vi "score target tracking.vi"() -> (0 "Boolean":bool)   [LabVIEW 2018]
uses:
  <vilib>/Rock Robotics/Network Tables/NT Write Number.vi
  <vilib>/Rock Robotics/Network Tables/NT Read Boolean.vi
  Robot Global Data.vi
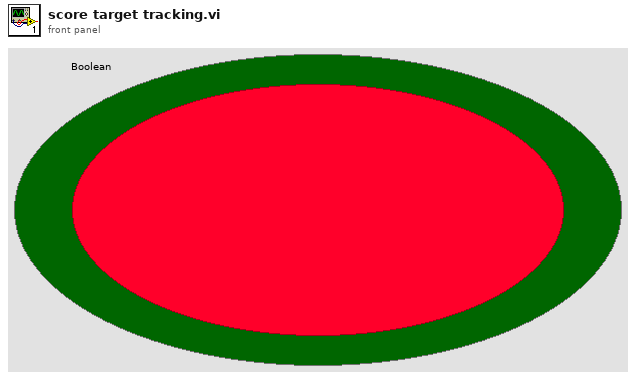
[diagram p1: front panel]
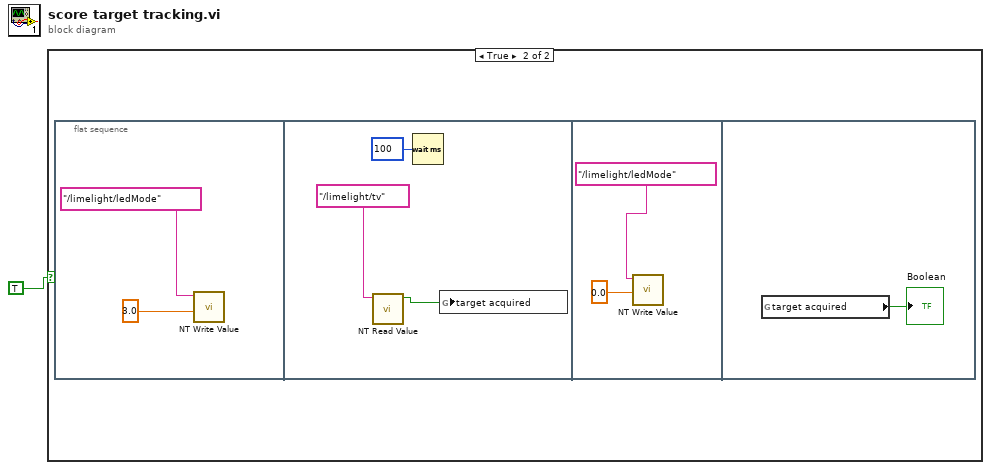
[diagram p0: block diagram]
diagram:
  n1 = case shown="True" TRUE {
    frame False {
    }
    frame True {
      n2 = flat-sequence {
        frame #0 {
          n3 = call-poly <vilib>:"NT Write Value.vi"("Numeric"=3.0, "Name"="/limelight/ledMode") -> ()  [unwired: 9 in, 1 out]
        }
        frame #1 {
          n4 = call-poly <vilib>:"NT Read Value.vi"("Name"="/limelight/tv") -> ("Boolean"=w5:bool)  [unwired: 9 in, 1 out]
          n5 = Wait (ms)(milliseconds to wait=u32 100) -> ()  [unwired: 1 out]
          n6 = global write "Robot Global Data.vi" "target acquired"(w5) -> ()
        }
        frame #2 {
          n7 = call-poly <vilib>:"NT Write Value.vi"("Numeric"=0.0, "Name"="/limelight/ledMode") -> ()  [unwired: 9 in, 1 out]
        }
        frame #3 {
          n8 = global read "Robot Global Data.vi" "target acquired"() -> (→"Boolean":bool)
        }
      }
    }
  }
